vi "Compile Function.vi"(8 "error in (no error)":errorcluster, 11 "functionbase in":refnum<class "functionbase.lvclass">) -> (0 "error out":errorcluster, 3 "functionbase out":refnum<class "functionbase.lvclass">)   [LabVIEW 2016, in "functionbase.lvclass"]
uses:
  functionbase.lvclass
  functionbase.lvclass/functionbase.ctl
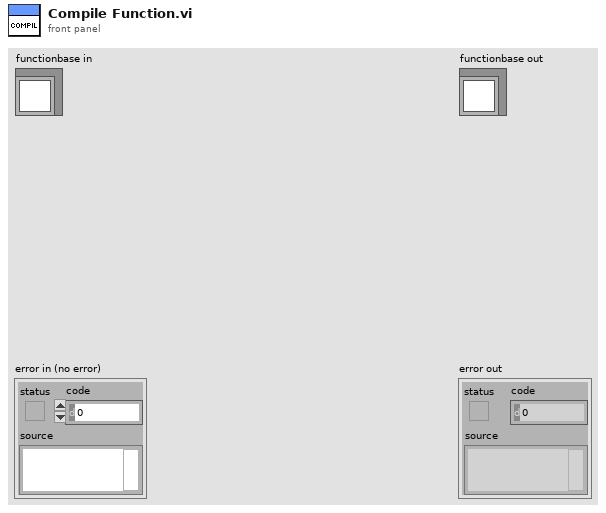
[diagram p1: front panel]
types:
  T1 = typedef "Scan Syntax Format.ctl" = cluster{"Syntax":string, "Variable#":i32, "Variables Name":string[]}
  T2 = typedef "Type Descriptor Enumeration__ogtk.ctl" = enum8{"<Null>", "I8", "I16", "I32", "I64", "U8", "U16", "U32", "U64", "SGL", "DBL", "EXT", "CSG", "CDB", "CXT", "0x0F", "0x10", "0x11", "0x12", "0x13", "0x14", "Enum U8", "Enum U16", "Enum U32", "Enum U64", "SGL PQ", "DBL PQ", "EXT PQ", "CSG PQ", "CDB PQ", "CXT PQ", "0x1F", "0x20", "Boolean", "0x22", "0x23", "0x24", "0x25", "0x26", "0x27", "0x28", "0x29", "0x2A", "0x2B", "0x2C", "0x2D", "0x2E", "0x2F", "String", "0x31", "Path", "Pict", "0x34", "0x35", "0x36", "DAQ", "0x38", "0x39", "0x3A", "0x3B", "0x3C", "0x3D", "0x3E", "0x3F", "Array", "0x41", "0x42", "0x43", "0x44", "0x45", "0x46", "0x47", "0x48", "0x49", "0x4A", "0x4B", "0x4C", "0x4D", "0x4E", "0x4F", "Cluster", "0x51", "0x52", "Variant", "Waveform", "0x55", "0x56", "0x57", "0x58", "0x59", "0x5A", "0x5B", "0x5C", "0x5D", "0x5E", "0x5F", "0x60", "0x61", "0x62", "0x63", "0x64", "0x65", "0x66", "0x67", "0x68", "0x69", "0x6A", "0x6B", "0x6C", "0x6D", "0x6E", "0x6F", "Refnum"}
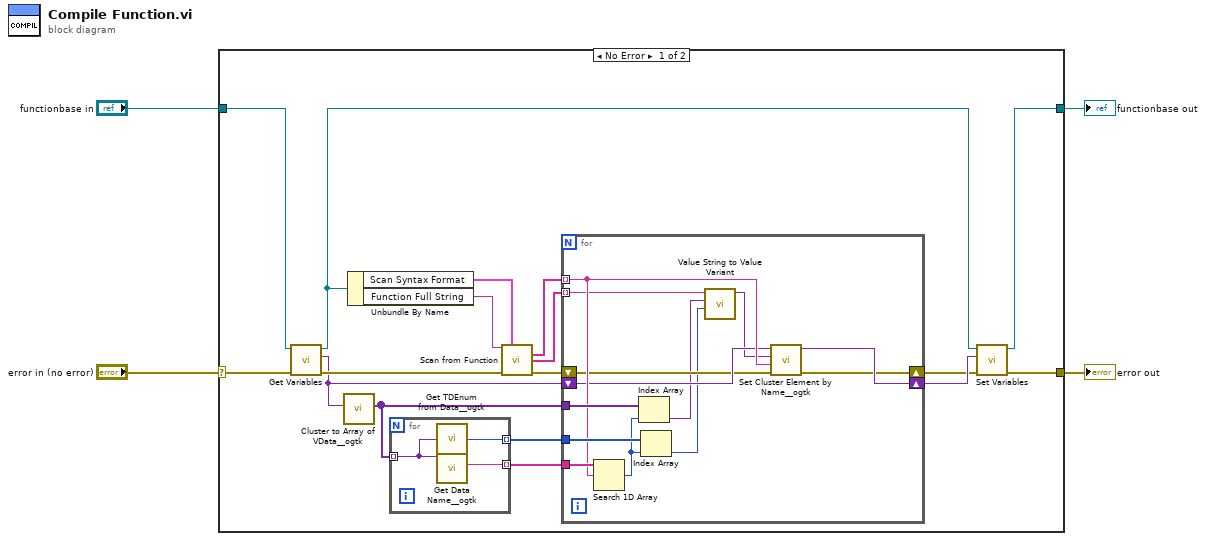
[diagram p0: block diagram]
diagram:
  n1 = case shown="No Error" "error in (no error)" {
    selector: "error in (no error)" -> [w21 w39]
    tunnel: [w19 w39] -> w3
    tunnel: [w18 w38] -> w1
    tunnel: "functionbase in" -> [w20 w38]
    frame No Error {
      n2 = call-dynamic "Get Variables.vi"("error in (no error)"=w21, "functionbase in"=w20) -> ("error out"=w17:errorcluster, "Variables"=w13:variant, "functionbase out"=w16:refnum<class "functionbase.lvclass">)  [unwired: 7 in]
      n3 = call <userlib>:"Cluster to Array of VData__ogtk.vi"("Cluster"=w13) -> ("Array of VData"=w11:variant[])  [unwired: 9 in, 1 out]
      n4 = Unbundle By Name(w16) -> ("Scan Syntax Format"=w14:T1, "Function Full String"=w15:string)
      n5 = for {
        tunnel: w11 -> [w37] mode=indexing
        tunnel: [w36] -> w10 mode=indexing
        tunnel: [w35] -> w9 mode=indexing
        n6 = call <userlib>:"Get TDEnum from Data__ogtk.vi"("Data"=w37) -> ("Type Descriptor Enumeration"=w36:T2)  [unwired: 4 in]
        n7 = call <userlib>:"Get Data Name__ogtk.vi"("Data"=w37) -> ("Data Name"=w35:string)  [unwired: 8 in, 2 out]
      }
      n8 = call "Scan from Function.vi"("initial string"=w15, "Syntax Format"=w14, "error in"=w17) -> ("Variables Name"=w8:string[], "Variables Value"=w7:string[], "error out"=w12:errorcluster)  [unwired: 9 in, 1 out]
      n9 = for {
        shift-right: [w29] -> w6
        shift-left: w13 -> [w28]
        shift-right: [w26] -> w5
        shift-left: w12 -> [w27]
        tunnel: w11 -> [w32]
        tunnel: w10 -> [w33]
        tunnel: w9 -> [w34]
        tunnel: w8 -> [w30] mode=indexing
        tunnel: w7 -> [w25] mode=indexing
        n10 = Search 1D Array(1D array=w34, element=w30) -> (index of element=w31:i32)  [unwired: 1 in]
        n11 = Index Array(array=w32, index=w31) -> (element=w22:variant)
        n12 = Index Array(array=w33, index=w31) -> (element=w23:T2)
        n13 = call "Value String to Value Variant.vi"("Type Descriptor Enumeration"=w23, "Default"=w22, "Value String"=w25) -> ("Value Variant"=w24:variant)  [unwired: 8 in]
        n14 = call <userlib>:"Set Cluster Element by Name__ogtk.vi"("error in (no error)"=w27, "Element Name (\"\": New Element Data Name)"=w30, "New Element Value"=w24, "Cluster"=w28) -> ("error out"=w26:errorcluster, "VCluster out"=w29:variant)  [unwired: 5 in, 1 out]
      }
      n15 = call-dynamic "Set Variables.vi"("error in (no error)"=w5, "Variables"=w6, "functionbase in"=w16) -> ("error out"=w19:errorcluster, "functionbase out"=w18:refnum<class "functionbase.lvclass">)  [unwired: 7 in]
    }
    frame Error {
    }
  }
  "error out" <- w3
  "functionbase out" <- w1
